vi "PROXY_parse_message_for_single_message_display.vi"(8 "error_in":errorcluster, 11 "message":string) -> (0 "error_out":errorcluster, 3 "parsed_message":string[][](array[string]))   [LabVIEW 2020]
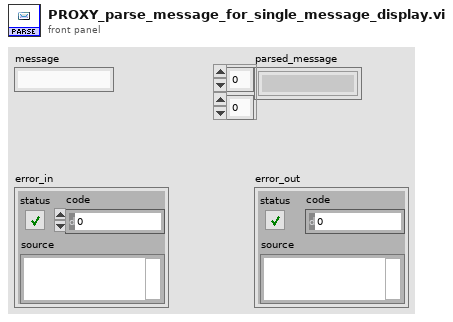
[diagram p1: front panel]
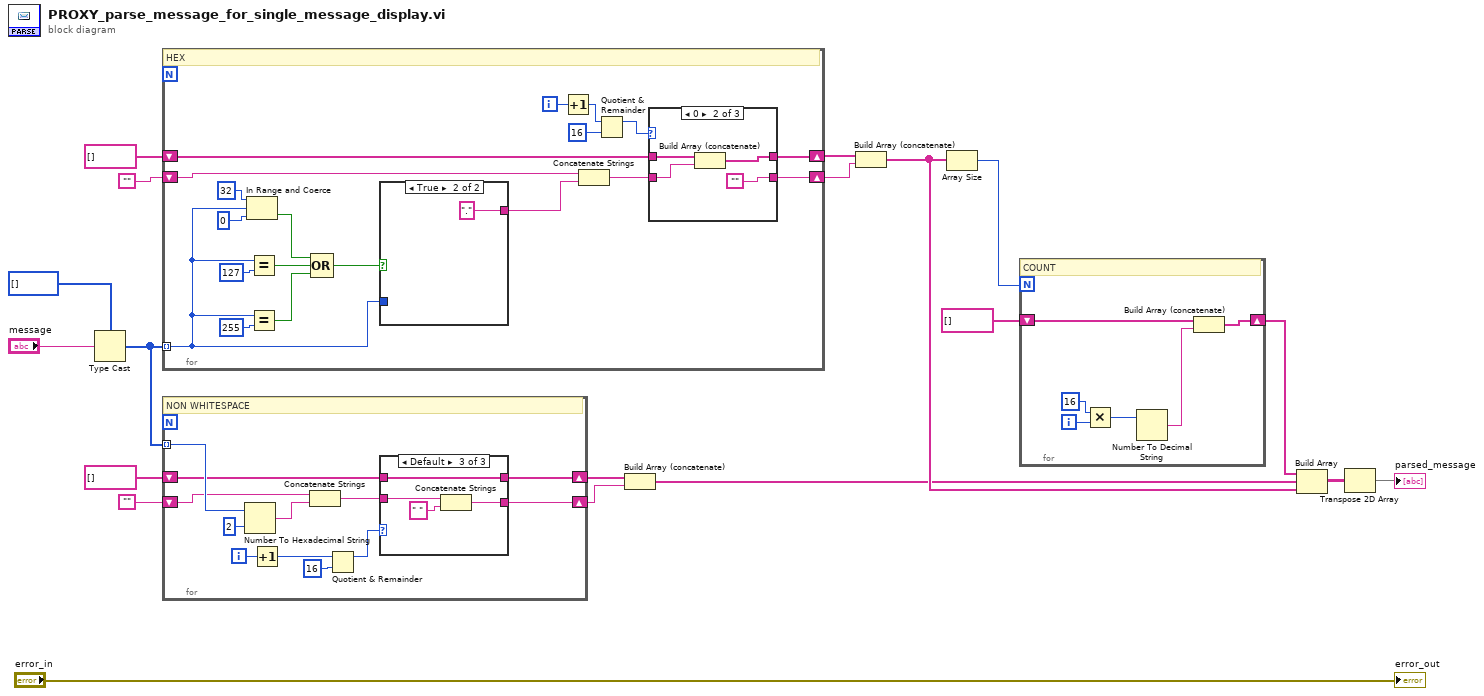
[diagram p0: block diagram]
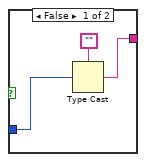
[diagram p2: hidden frame]
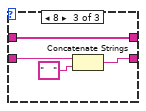
[diagram p4: hidden frame]
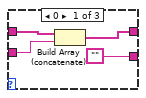
[diagram p5: hidden frame]
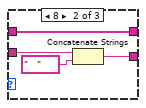
[diagram p6: hidden frame]
diagram:
  n1 = Type Cast(type=u8[] [], x="message") -> (*(type *) &x=w14:u8[])
  n2 = for {
    tunnel: w14 -> [w26] mode=indexing
    shift-right: [w21] -> w6
    shift-left: string[] [] -> [w22]
    shift-right: [w20] -> w5
    shift-left: "" -> [w24]
    i -> [w29]
    # "HEX"
    n3 = In Range and Coerce(upper limit=u8 32, x=w26, lower limit=u8 0) -> (In Range?=w36:bool)  [unwired: 1 out]
    n4 = Equal?(x=w26, y=u8 127) -> (x = y?=w33:bool)
    n5 = Equal?(x=w26, y=u8 255) -> (x = y?=w32:bool)
    n6 = Compound Arithmetic op=OR(w36, w33, w32) -> (w27:bool)
    n7 = case shown="True" w27 {
      tunnel: w26 -> [w40 _]
      tunnel: [w39 "."] -> w25
      frame False {
        n8 = Type Cast(type="", x=w40) -> (*(type *) &x=w39:string)
      }
      frame True {
      }
    }
    n9 = Increment(x=w29) -> (x+1=w31:i32)
    n10 = Concatenate Strings(w24, w25) -> (w23:string)
    n11 = Quotient & Remainder(x=w31, y=16) -> (x-y*floor(x/y)=w28:i32)  [unwired: 1 out]
    n12 = case shown="0" w28 {
      tunnel: w23 -> [w43 w47 w50]
      tunnel: w22 -> [w44 w48 w52]
      tunnel: [w44 w46 w52] -> w21
      tunnel: [w43 "" w49] -> w20
      frame Default {
      }
      frame 0 {
        n13 = Build Array (concatenate)(w48, w47) -> (w46:string[])
      }
      frame 8 {
        n14 = Concatenate Strings(w50, "   " ("string")) -> (w49:string)
      }
    }
  }
  n15 = for {
    tunnel: w14 -> [w63] mode=indexing
    shift-right: [w58] -> w3
    shift-left: "" -> [w62]
    shift-right: [w53] -> w2
    shift-left: string[] [] -> [w54]
    i -> [w56]
    # "NON WHITESPACE"
    n16 = Number To Hexadecimal String(1:i16 2 ("width (-)"), 2:w63) -> (0:w61:string)
    n17 = Increment(x=w56) -> (x+1=w55:i32)
    n18 = Concatenate Strings(w62, w61) -> (w59:string)
    n19 = Quotient & Remainder(x=w55, y=16) -> (x-y*floor(x/y)=w57:i32)  [unwired: 1 out]
    n20 = case shown="Default" w57 {
      tunnel: w59 -> [w67 w72 w76]
      tunnel: ["" w71 w75] -> w58
      tunnel: w54 -> [w68 w69 w73]
      tunnel: [w66 w69 w73] -> w53
      frame 0 {
        n21 = Build Array (concatenate)(w68, w67) -> (w66:string[])
      }
      frame 8 {
        n22 = Concatenate Strings(w72, "   " ("string")) -> (w71:string)
      }
      frame Default {
        n23 = Concatenate Strings(w76, " " ("string")) -> (w75:string)
      }
    }
  }
  n24 = Build Array (concatenate)(w2, w3) -> (w1:string[])
  n25 = Build Array (concatenate)(w6, w5) -> (w4:string[])
  n26 = Array Size(array=w4) -> (size(s)=w18:i32)
  n27 = for {
    N: w18 -> [_]
    shift-right: [w77] -> w19
    shift-left: string[] [] -> [w78]
    i -> [w82]
    # "COUNT"
    n28 = Multiply(x=16, y=w82) -> (x*y=w80:i32)
    n29 = Number To Decimal String(number=w80) -> (decimal integer string=w79:string)  [unwired: 1 in]
    n30 = Build Array (concatenate)(w78, w79) -> (w77:string[])
  }
  n31 = Build Array(w19, w1, w4) -> (w8:string[][])
  n32 = Transpose 2D Array(2D array=w8) -> (transposed array=→"parsed_message":string[][])
  "error_out" <- "error_in"
